vi "VI Set Debugging.vi"(8 "error in (no error)":errorcluster, 10 "Allow Debugging":bool, 11 "vi ref in":refnum<vi>) -> (0 "error out":errorcluster, 3 "vi ref out":refnum<vi>)   [LabVIEW 2017, in "Build Automation.lvlib"]
uses:
  Build Automation.lvlib
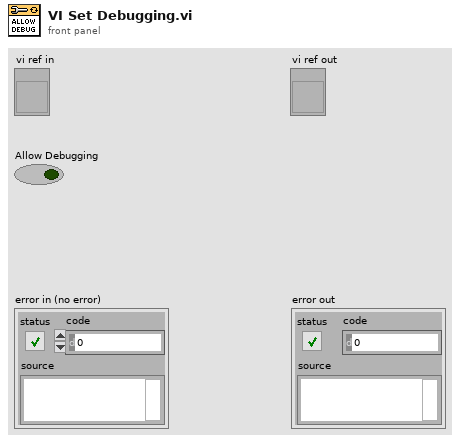
[diagram p1: front panel]
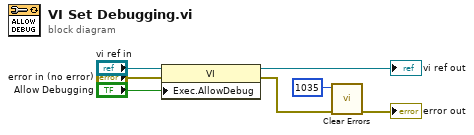
[diagram p0: block diagram]
diagram:
  n1 = property class="VI"(reference="vi ref in", error in="error in (no error)", "Exec.AllowDebug"="Allow Debugging") -> (reference out=→"vi ref out":refnum<vi>, error out=w2:errorcluster)
  n2 = call <vilib>:"Clear Errors.vi"("error in (no error)"=w2, "specific error code to clear (0: all)"=1035) -> ("error out"=→"error out":errorcluster)  [unwired: 4 in, 1 out]
